vi "GCentral Website Root URL--constant.vi"() -> (3 "Website Root URL":string="https://intranet.studiobods.com/public/temp/GCentral/PackageDetails.html")   [LabVIEW 2016, in "WSsupport.lvlib"]
uses:
  WSsupport.lvlib
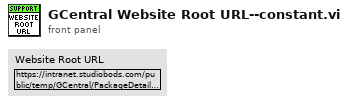
[diagram p1: front panel]
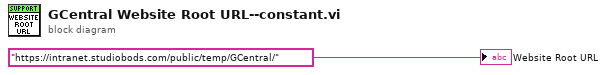
[diagram p0: block diagram]
diagram:
  "Website Root URL" <- "https://intranet.studiobods.com/public/temp/GCentral/"
